vi "Set VI Ref.vi"(8 "error in":errorcluster, 10 "VI Refnum":refnum<vi>, 11 "Class in":refnum<class>) -> (0 "error out":errorcluster, 3 "Class out":refnum<class>)   [LabVIEW 2023, in "Label-Driven UI.lvlib"]
doc: "입력한 클래스와 그 클래스에서 UI를 담당하는 VI의 참조를 매칭하여, 다른 메소드를 사용할 때 이 클래스 정보와 참조를 이용합니다."
uses:
  Label-Driven UI.lvlib
  Map Cmd.ctl
  <vilib>/Utility/error.llb/Error Cluster From Error Code.vi
  <vilib>/ErrorRing/Error Ring.xnode
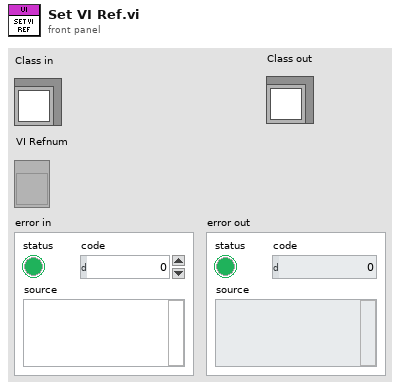
[diagram p1: front panel]
types:
  T1 = typedef "Label-Driven UI.lvlib/Map Cmd.ctl" = enum16{"Insert", "Delete", "Look"}
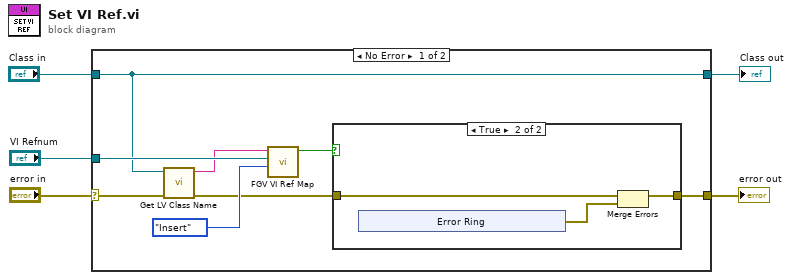
[diagram p0: block diagram]
diagram:
  n1 = case shown="No Error" "error in" {
    selector: "error in" -> [w7 w23]
    tunnel: "Class in" -> [w9 w24]
    tunnel: [w11 w23] -> w3
    tunnel: [w9 w24] -> w2
    tunnel: "VI Refnum" -> [w10 _]
    frame No Error {
      n2 = call <vilib>:"Get LV Class Name.vi"("error in (no error)"=w7, "object"=w9) -> ("error out"=w6:errorcluster, "class name"=w8:string)  [unwired: 8 in]
      n3 = call "FGV VI Ref Map.vi"("Map Cmd"=Map_Cmd."Insert", "VI Ref in"=w10, "Class Name"=w8) -> ("isExist"=w12:bool)  [unwired: 7 in, 1 out]
      n4 = case shown="True" w12 {
        tunnel: w6 -> [w14 w16]
        tunnel: [w14 w15] -> w11
        frame False {
        }
        frame True {
          n5 = xnode "Error Ring"() -> ("error out"=w17:errorcluster)
          n6 = Merge Errors(w16, w17) -> (w15:errorcluster)
        }
      }
    }
    frame Error {
    }
  }
  "Class out" <- w2
  "error out" <- w3
